vi "random-timesig.vi"(11 "appended array":i32[][](array[numeric])) -> (1 "String":string, 2 "Numeric":i32, 3 "output array":i32[][](array[numeric]))   [LabVIEW 2019]
uses:
  <vilib>/numeric/Random Number (Range) I64.vi
  <vilib>/numeric/sub_Random U32.vi
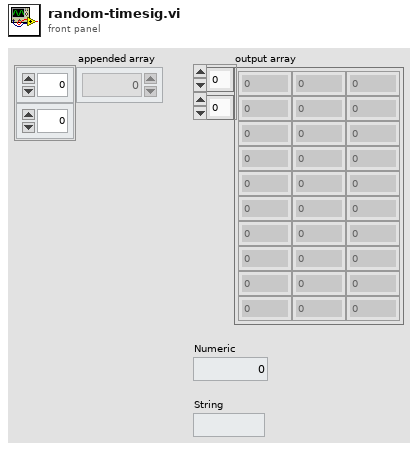
[diagram p1: front panel]
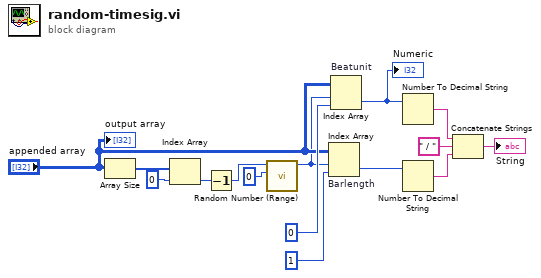
[diagram p0: block diagram]
diagram:
  n1 = Array Size(array="appended array") -> (size(s)=w5:i32[])
  n2 = Index Array(array=w5, index=0) -> (element=w4:i32)
  n3 = Decrement(x=w4) -> (x-1=w1:i32)
  n4 = call-poly <vilib>:"Random Number (Range).vi"("lower bound (-100)"=i64 0, "upper bound (100)"=w1) -> ("number"=w3:i64)  [unwired: 9 in]
  n5 = Index Array "Barlength"(array="appended array", index (row)=w3, index (col)=1 ("disabled index (col)")) -> (element=w10:i32)
  n6 = Index Array "Beatunit"(array="appended array", index (row)=w3, index (col)=0 ("disabled index (col)")) -> (element=w15:i32)
  "Numeric" <- w15
  n7 = Number To Decimal String(number=w15) -> (decimal integer string=w11:string)  [unwired: 1 in]
  n8 = Number To Decimal String(number=w10) -> (decimal integer string=w13:string)  [unwired: 1 in]
  n9 = Concatenate Strings(w11, " / " ("string"), w13) -> (→"String":string)
  "output array" <- "appended array"
